vi "set_pid_high_clamping_limit.vi"(8 "error in (no error)":errorcluster, 10 "High clamping limit (%)":i32, 11 "connection ID":refnum<k5>) -> (0 "error out":errorcluster, 3 "connection ID out":refnum<k5>)   [LabVIEW 2018]
panel:
  out "bytes written":i32
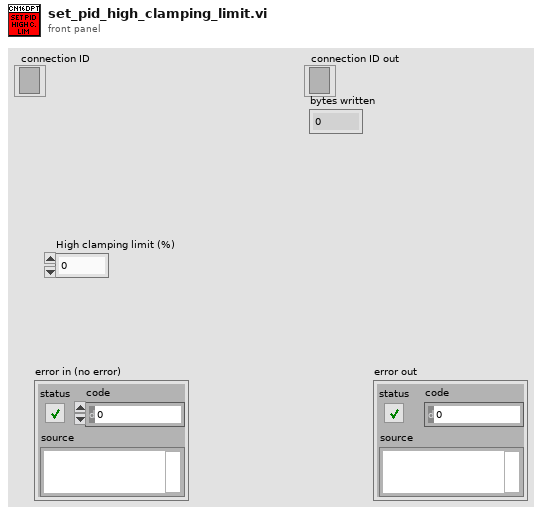
[diagram p1: front panel]
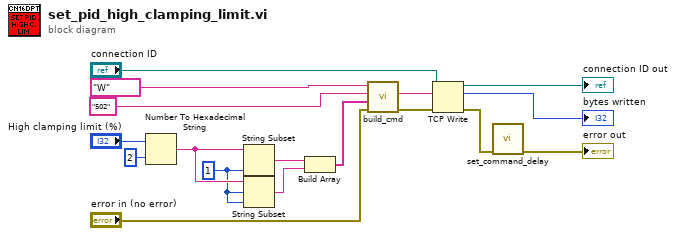
[diagram p0: block diagram]
diagram:
  w10 = 1 ("length (rest)")
  n1 = Number To Hexadecimal String(1:i16 2 ("width (-)"), 2:"High clamping limit (%)") -> (0:w11:string)
  n2 = String Subset(string=w11, length (rest)=w10) -> (substring=w9:string)  [unwired: 1 in]
  n3 = String Subset(string=w11, offset (0)=w10, length (rest)=w10) -> (substring=w8:string)
  n4 = Build Array(w9, w8) -> (w7:string[])
  n5 = call "build_cmd.vi"("error in (no error)"="error in (no error)", "Parameter list"=w7, "Command ID"="502", "Command class"="W") -> ("error out"=w14:errorcluster, "Command"=w13:string)  [unwired: 6 in]
  n6 = TCP Write(connection ID="connection ID", data in=w13, error in (no error)=w14) -> (connection ID out=→"connection ID out":refnum<k5>, bytes written=→"bytes written":i32, error out=w3:errorcluster)  [unwired: 1 in]
  n7 = call "set_command_delay.vi"("error in (no error)"=w3) -> ("error out"=→"error out":errorcluster)  [unwired: 10 in]
